vi "close shutter.vi"(8 "error in (no error)":errorcluster, 11 "Murmex in":refnum<class "Murmex.lvclass">) -> (0 "error out":errorcluster, 3 "Murmex out":refnum<class "Murmex.lvclass">)   [LabVIEW 2012]
uses:
  <vilib>/Distrio/Murmex/Murmex/Murmex.lvclass
  <vilib>/Distrio/Murmex/GenericMessage/GenericMessage.lvclass
  <vilib>/Distrio/Murmex/Message/Add or replace parameter.vi
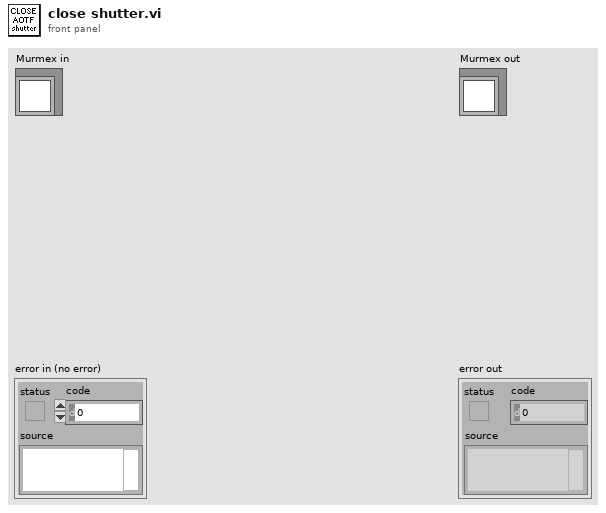
[diagram p1: front panel]
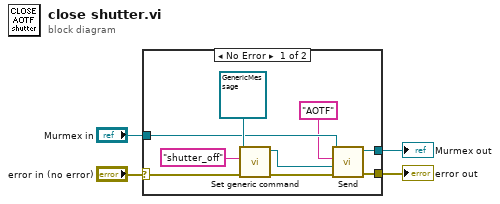
[diagram p0: block diagram]
diagram:
  n1 = case shown="No Error" "error in (no error)" {
    selector: "error in (no error)" -> [w7 w15]
    tunnel: [w13 w15] -> w3
    tunnel: [w12 w14] -> w1
    tunnel: "Murmex in" -> [w6 w14]
    frame No Error {
      n2 = call <vilib>:"Set generic command.vi"("error in (no error)"=w7, "generic command"="shutter_off", "GenericMessage in"=refnum<class "GenericMessage.lvclass"> refnum ("Murmex.lvlib:GenericMessage")) -> ("error out"=w10:errorcluster, "GenericMessage out"=w9:refnum<class "GenericMessage.lvclass">)  [unwired: 7 in]
      n3 = call <vilib>:"Send.vi"("error in (no error)"=w10, "Message"=w9, "recipient"="AOTF", "Murmex in"=w6) -> ("error out"=w13:errorcluster, "Murmex out"=w12:refnum<class "Murmex.lvclass">)  [unwired: 6 in]
    }
    frame Error {
    }
  }
  "error out" <- w3
  "Murmex out" <- w1
